vi "Mandelbrot.vi"() -> ()   [LabVIEW 2018]
panel:
  out "XY Graph":cluster{"Y":dbl[], "Y":dbl[]}[](graph)
  in  "number of points along one axis":i32=500
  in  "y max":dbl=2.0
  in  "y min":dbl=-2.0
  in  "x max":dbl=2.0
  in  "x min":dbl=-2.0
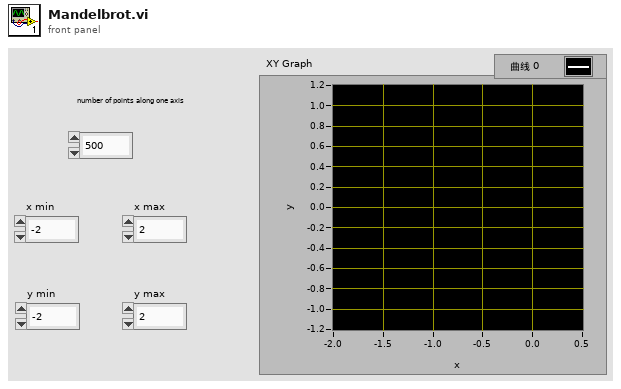
[diagram p1: front panel]
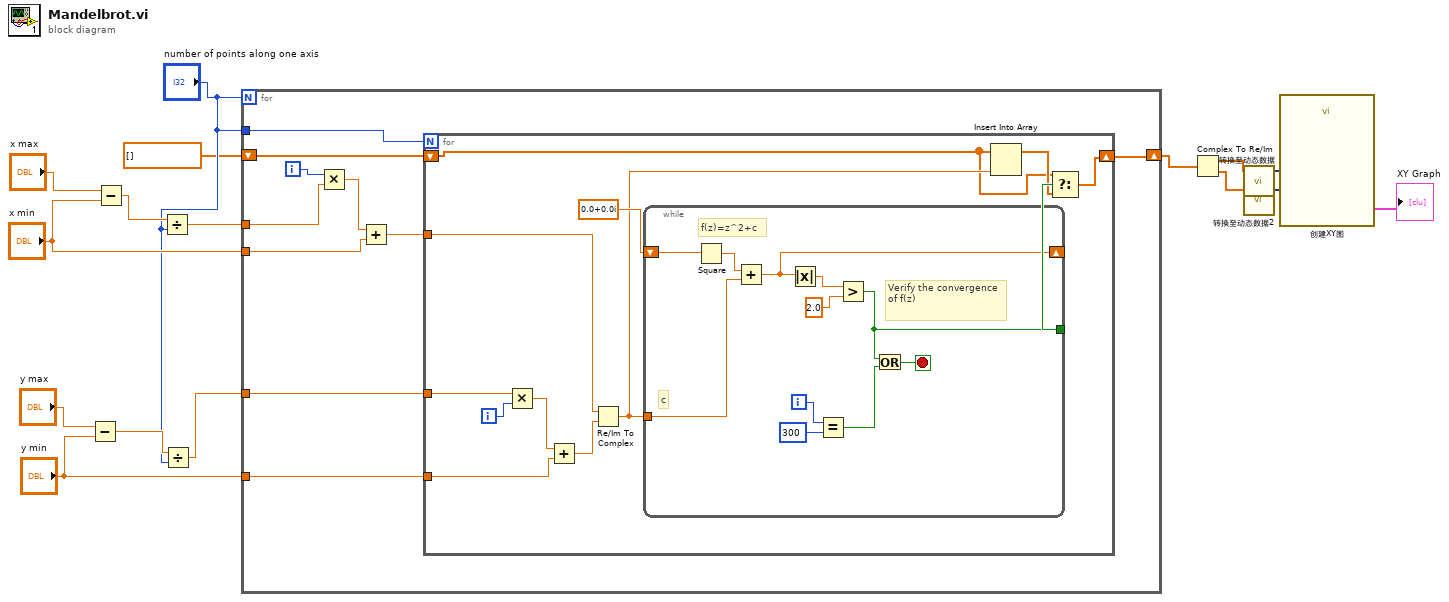
[diagram p0: block diagram]
diagram:
  n1 = Subtract(x="y max", y="y min") -> (x-y=w13:dbl)
  n2 = Subtract(x="x max", y="x min") -> (x-y=w14:dbl)
  n3 = Divide(x=w14, y="number of points along one axis") -> (x/y=w12:dbl)
  n4 = Divide(x=w13, y="number of points along one axis") -> (x/y=w9:dbl)
  n5 = for {
    N: "number of points along one axis" -> [_]
    tunnel: w12 -> [w26]
    tunnel: "x min" -> [w23]
    tunnel: "number of points along one axis" -> [w22]
    tunnel: w9 -> [w21]
    tunnel: "y min" -> [w20]
    shift-right: [w17] -> w6
    shift-left: cdb[] [] ("数组") -> [w18]
    i -> [w25]
    n6 = Multiply(x=w25, y=w26) -> (x*y=w24:dbl)
    n7 = Add(x=w24, y=w23) -> (x+y=w19:dbl)
    n8 = for {
      N: w22 -> [_]
      tunnel: w21 -> [w36]
      tunnel: w20 -> [w35]
      tunnel: w19 -> [w33]
      shift-right: [w29] -> w17
      shift-left: w18 -> [w27]
      i -> [w37]
      n9 = Multiply(x=w36, y=w37) -> (x*y=w38:dbl)
      n10 = Add(x=w38, y=w35) -> (x+y=w34:dbl)
      n11 = Re/Im To Complex(1:w34, 2:w33) -> (0:w30:cdb)
      n12 = while {
        tunnel: w30 -> [w49]
        shift-right: [w46] -> _
        shift-left: cdb 0.0+0.0i ("x") -> [w47]
        tunnel: [w39] -> w31
        i -> [w45]
        stop <- w43 stop-if-true
        # "Verify the convergence of f(z)"
        # "f(z)=z^2+c"
        # "c"
        n13 = Square(x=w47) -> (x^2=w48:cdb)
        n14 = Add(x=w48, y=w49) -> (x+y=w46:cdb)
        n15 = Absolute Value(x=w46) -> (abs(x)=w41:dbl)
        n16 = Equal?(x=w45, y=300) -> (x = y?=w42:bool)
        n17 = Greater?(x=w41, y=2.0) -> (0:w39:bool)
        n18 = Or(x=w39, y=w42) -> (x .or. y?=w43:bool)
      }
      n19 = Insert Into Array(array=w27, new element=w30) -> (w28:cdb[])  [unwired: 1 in]
      n20 = Select(t=w27, s=w31, f=w28) -> (s? t:f=w29:cdb[])
    }
  }
  n21 = Complex To Re/Im(x + iy=w6) -> (x=w4:dbl[], y=w2:dbl[])
  n22 = call "转换至动态数据"("Array"=w4) -> ("Dynamic Data Type"=w3:dynamicdata)  [unwired: 3 in]
  n23 = call "转换至动态数据2"("Array"=w2) -> ("Dynamic Data Type"=w1:dynamicdata)  [unwired: 3 in]
  n24 = call "创建XY图"("Y Input"=w1, "X Input"=w3) -> ("XY Graph"=→"XY Graph":cluster{"X":dbl[], "Y":dbl[]}[])  [unwired: 8 in, 1 out]
